vi "Read Enable Output Command (Array).vi"(8 "error in":errorcluster, 11 "Power Supply in":refnum<class "Power Supply.lvclass">) -> (0 "error out":errorcluster, 1 "Changed or First Call?":bool, 2 "Enable Output":bool[](array[boolean]), 3 "Power Supply out":refnum<class "Power Supply.lvclass">)   [LabVIEW 2023, in "Power Supply.lvclass"]
uses:
  Power Supply.lvclass
  Power Supply.lvclass/Power Supply.ctl
  <vilib>/ADAS Replay HIL/Channels/Tag Wrapper/Polymorphic/Read Channel (Boolean).vi
  28ca3c79-95f5-44c6-ac38-ea14683abb8a.vi
  <vilib>/ADAS Replay HIL/Channels/Tag Wrapper/Polymorphic/Read Channel (Boolean).vi/b2f764de-0c1e-4784-a155-687fc995a684.vi
  <vilib>/ADAS Replay HIL/Channels/Tag Wrapper/Polymorphic/Read Channel (Boolean).vi/b2f764de-0c1e-4784-a155-687fc995a684.vi/c28b0ead-42ad-4072-80a2-aca7f2bd7ce3.vi
  <vilib>/ADAS Replay HIL/Channels/Tag Wrapper/Polymorphic/Read Channel (Boolean).vi/b2f764de-0c1e-4784-a155-687fc995a684.vi/219d0231-d98b-4193-b5cc-84f90e3c9091.vi
  <vilib>/ADAS Replay HIL/Channels/Tag Wrapper/Tag Wrapper.lvlib
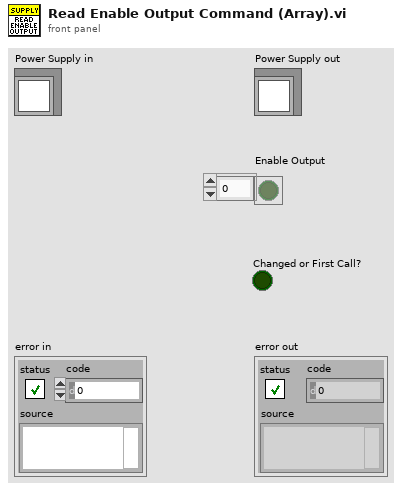
[diagram p1: front panel]
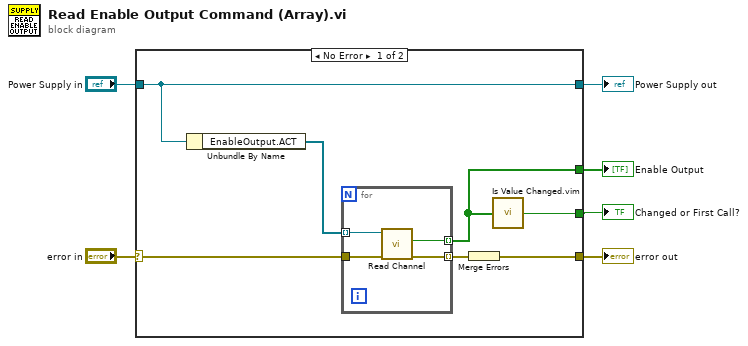
[diagram p0: block diagram]
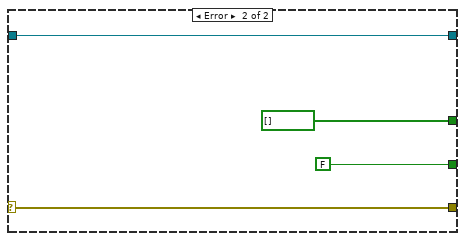
[diagram p2: hidden frame]
diagram:
  n1 = case shown="No Error" "error in" {
    selector: "error in" -> [w12 w20]
    tunnel: [w9 w20] -> w5
    tunnel: [w13 w21] -> w3
    tunnel: "Power Supply in" -> [w13 w21]
    tunnel: [w8 bool[] []] -> w2
    tunnel: [w7 FALSE ("changed or first call?")] -> w1
    frame No Error {
      n2 = Unbundle By Name(w13) -> ("EnableOutput.ACT"=w10:refnum<k21>[])
      n3 = for {
        tunnel: w10 -> [w15] mode=indexing
        tunnel: [w14] -> w8 mode=indexing
        tunnel: w12 -> [w17]
        tunnel: [w16] -> w11 mode=indexing
        n4 = call-poly <vilib>:"Read Channel.vi"("error in"=w17, "ADAS HIL Channel in"=w15) -> ("error out"=w16:errorcluster, "Value out"=w14:bool)  [unwired: 6 in, 2 out]
      }
      n5 = Merge Errors(w11) -> (w9:errorcluster)
      n6 = call "Is Value Changed.vim"("value"=w8) -> ("changed or first call?"=w7:bool)
    }
    frame Error {
    }
  }
  "error out" <- w5
  "Power Supply out" <- w3
  "Enable Output" <- w2
  "Changed or First Call?" <- w1
